vi "dispatchTask.vi"(0 "HGF_ThreadPool_Reference":refnum<class "HGF_Reference.lvclass">, 2 "HGF_ThreadTask":refnum<class "HGF_ThreadTask.lvclass">, 3 "timeout in ms (-1)":i32=-1, 5 "error in (no error)":errorcluster) -> (14 "dup HGF_ThreadPool_Reference":refnum<class "HGF_Reference.lvclass">, 17 "got object?":bool, 19 "error out":errorcluster)   [LabVIEW 2014, in "HGF_BaseClasses.lvlib" / "HGF_ThreadPool.lvclass"]
doc: "Start new threads."
uses:
  HGF_ThreadPool.lvclass
  HGF_Reference/HGF_Reference.lvclass
  HGF_ThreadTask/HGF_ThreadTask.lvclass
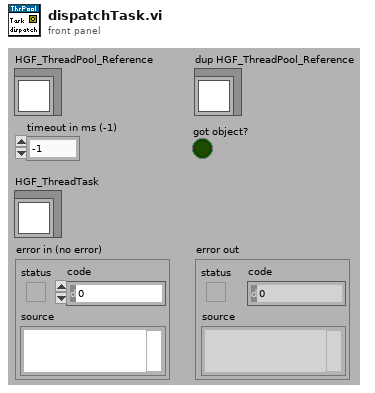
[diagram p1: front panel]
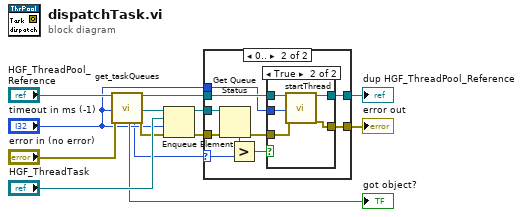
[diagram p0: block diagram]
diagram:
  n1 = call "get_taskQueues.vi"("HGF_ThreadPool_Reference"="HGF_ThreadPool_Reference", "timeout in ms (-1)"="timeout in ms (-1)", "error in (no error)"="error in (no error)") -> ("got object?"=→"got object?":bool, "autoIncrementLimit"=w1:i32, "dup HGF_ThreadPool_Reference"=w5:refnum<class "HGF_Reference.lvclass">, "taskQueue in"=w12:refnum<queue>, "error out"=w10:errorcluster)  [unwired: 12 out]
  n2 = Enqueue Element(queue=w12, element="HGF_ThreadTask", timeout in ms (-1)="timeout in ms (-1)", error in (no error)=w10) -> (queue out=w8:refnum<queue>, error out=w7:errorcluster)  [unwired: 1 out]
  n3 = case shown="0.." w1 {
    selector: w1 -> [_ w16]
    tunnel: w8 -> [_ w25]
    tunnel: w7 -> [w14 w24]
    tunnel: w5 -> [w15 w22]
    tunnel: [w15 w20] -> w4
    tunnel: [w14 w19] -> w3
    tunnel: "timeout in ms (-1)" -> [_ w18]
    frame Default {
    }
    frame 0.. {
      n4 = Get Queue Status(queue=w25, error in (no error)=w24) -> (error out=w21:errorcluster, # elements in queue=w23:i32)  [unwired: 7 out]
      n5 = Greater?(x=w23, y=w16) -> (0:w17:bool)
      n6 = case shown="True" w17 {
        tunnel: w22 -> [w27 w32]
        tunnel: w21 -> [w26 w31]
        tunnel: w18 -> [_ w30]
        tunnel: [w27 w29] -> w20
        tunnel: [w26 w28] -> w19
        frame False {
        }
        frame True {
          n7 = call "startThread.vi"("HGF_ThreadPool_Reference"=w32, "timeout in ms (-1)"=w30, "error in (no error)"=w31) -> ("dup HGF_ThreadPool_Reference"=w29:refnum<class "HGF_Reference.lvclass">, "error out"=w28:errorcluster)  [unwired: 15 out]
        }
      }
    }
  }
  "error out" <- w3
  "dup HGF_ThreadPool_Reference" <- w4
